vi "TEST Data processing.vi"() -> ()   [LabVIEW 2017]
uses:
  <vilib>/measure/mascope.llb/Pulse Measurements 1 chan.vi
  <vilib>/DAQmx/read.llb/DAQmx Read (Digital Wfm 1Chan NSamp Duration).vi
  <vilib>/measure/NI_MAPro.lvlib
  <vilib>/measure/NI_MABase.lvlib
panel:
  in  "sampling info":cluster{"Fs":dbl, "#s":dbl}={"Fs"=1000.0, "#s"=1000.0} {"Fs" format="%.2p"}
  out "Waveform Graph":waveform(dbl)(graph)
  in  "frequency":dbl=10.0
  out "1/x 2":dbl
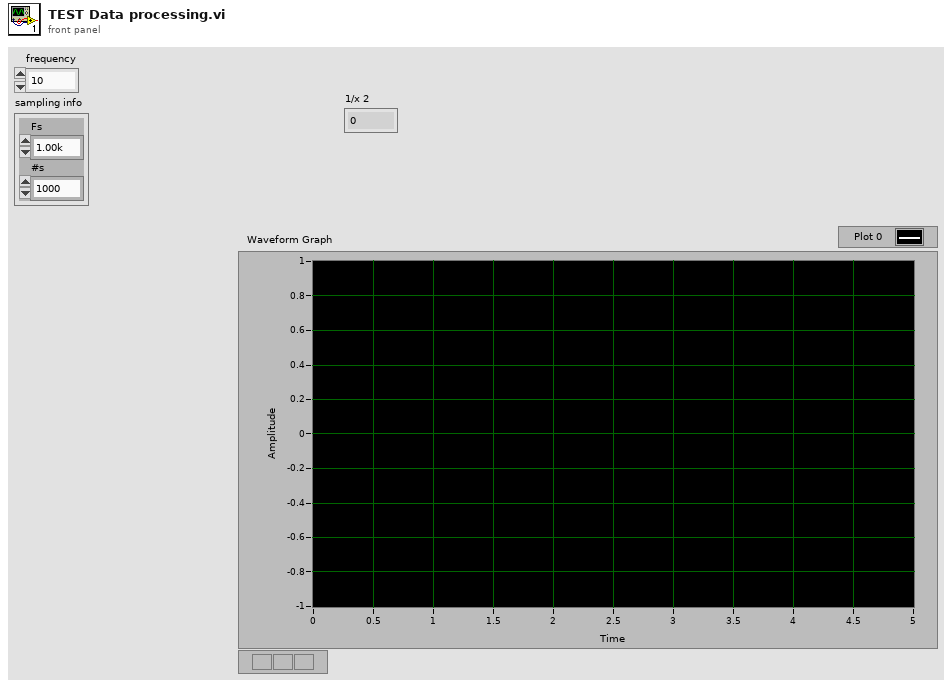
[diagram p1: front panel]
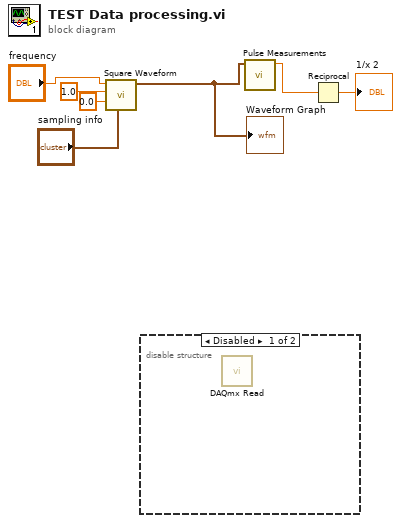
[diagram p0: block diagram]
diagram:
  n1 = call <vilib>:"Square Waveform.vi"("sampling info"="sampling info", "phase"=0.0, "amplitude"=1.0, "frequency"="frequency") -> ("signal out"=w2:waveform(dbl))  [unwired: 6 in, 1 out]
  "Waveform Graph" <- w2
  n2 = disable-structure shown="Disabled" {
    frame Disabled {
      n3 = call-poly <vilib>:"DAQmx Read.vi"() -> ()  [unwired: 13 in, 3 out]
    }
    frame Enabled {
    }
  }
  n4 = call-poly <vilib>:"Pulse Measurements.vi"("signal in"=w2) -> ("period"=w5:dbl)  [unwired: 6 in, 4 out]
  n5 = Reciprocal(x=w5) -> (1/x=→"1/x 2":dbl)
